vi "ExecuteSkill.vi"(0 "object in":refnum<class "AlignSkill.lvclass">, 2 "Robot in":refnum<class "Robot.lvclass">, 4 "GameRef":refnum<data-value>, 5 "error in (no error)":errorcluster) -> (14 "object out":refnum<class "AlignSkill.lvclass">, 16 "Robot out":refnum<class "Robot.lvclass">, 19 "error out":errorcluster)   [LabVIEW 2023, in "AlignSkill.lvclass"]
uses:
  AlignSkill.lvclass
  Robot_class/Robot.lvclass
  Game_class/Game.lvclass
  GoToSkill_v2_class/GoToSkill_v2.lvclass
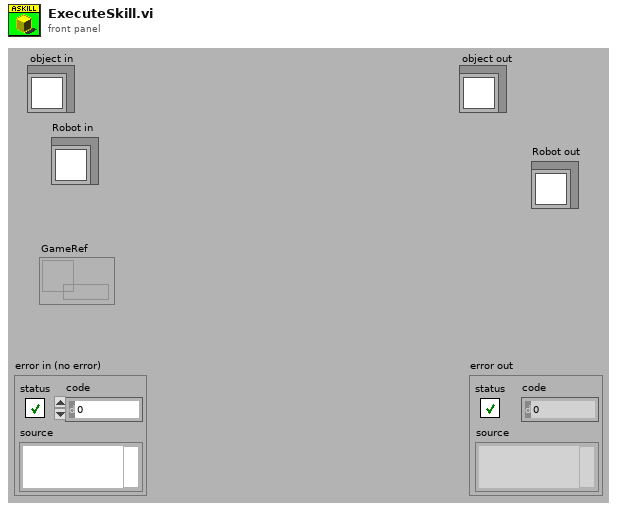
[diagram p1: front panel]
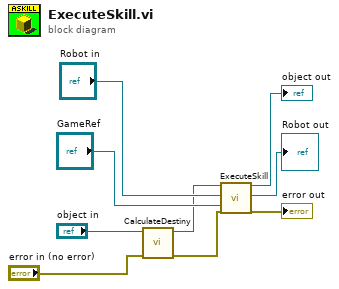
[diagram p0: block diagram]
diagram:
  n1 = call-dynamic "CalculateDestiny.vi"("error in (no error)"="error in (no error)", "AlignSkill in"="object in") -> ("error out"=w1:errorcluster, "AlignSkill out"=w3:refnum<class "AlignSkill.lvclass">)  [unwired: 8 in]
  n2 = call-parent "ExecuteSkill.vi"("object in"=w3, "Robot in"="Robot in", "GameRef"="GameRef", "error in (no error)"=w1) -> ("object out"=→"object out":refnum<class "AlignSkill.lvclass">, "Robot out"=→"Robot out":refnum<class "Robot.lvclass">, "error out"=→"error out":errorcluster)  [unwired: 13 in]
